vi "set voltage.vi"(8 "error in (no error)":errorcluster, 10 "Voltage":dbl, 11 "BK 9202B in":refnum<class "BK 9202B.lvclass">) -> (0 "error out":errorcluster, 3 "BK 9202B out":refnum<class "BK 9202B.lvclass">)   [LabVIEW 2025, in "Power Supply.lvlib" / "BK 9202B.lvclass"]
uses:
  BK 9202B.lvclass
  BK 9202B.lvclass/BK 9202B.ctl
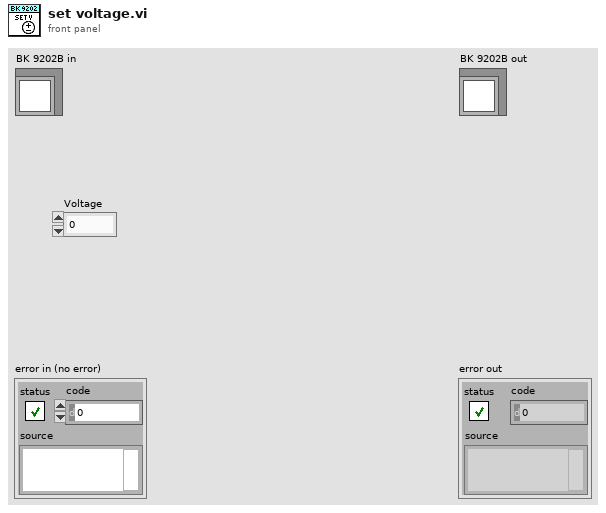
[diagram p1: front panel]
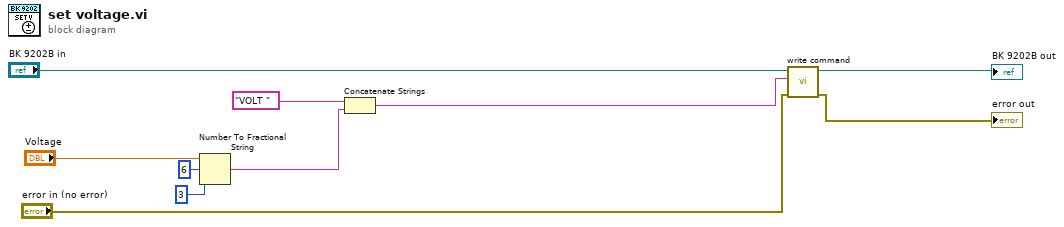
[diagram p0: block diagram]
diagram:
  n1 = Number To Fractional String(number="Voltage", width (-)=i16 6, precision (6)=i16 3) -> (F-format string=w3:string)  [unwired: 1 in]
  n2 = Concatenate Strings("VOLT ", w3) -> (w2:string)
  n3 = call "write command.vi"("error in (no error)"="error in (no error)", "string"=w2, "BK 9202B in"="BK 9202B in") -> ("error out"=→"error out":errorcluster, "BK 9202B out"=→"BK 9202B out":refnum<class "BK 9202B.lvclass">)  [unwired: 7 in]
